vi "Check Notebook Status Before Quitting App.vi"(8 "Error In":errorcluster, 11 "App name":string) -> (0 "Error Out":errorcluster, 3 "Quit App?":bool)   [LabVIEW 2021, in "Notebook.lvlib"]
uses:
  Notebook.lvlib
  Notebook Parameters List.ctl
  Variant/Variant to Data/Variant to Data.lvlib
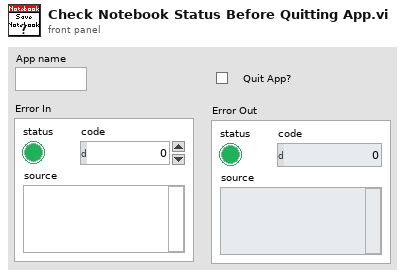
[diagram p1: front panel]
types:
  T1 = typedef "Notebook.lvlib/Notebook Parameters List.ctl" = enum16{"First Opening?", "Saved Notebook?", "Saved Notebook Path", "Beep on Error?"}
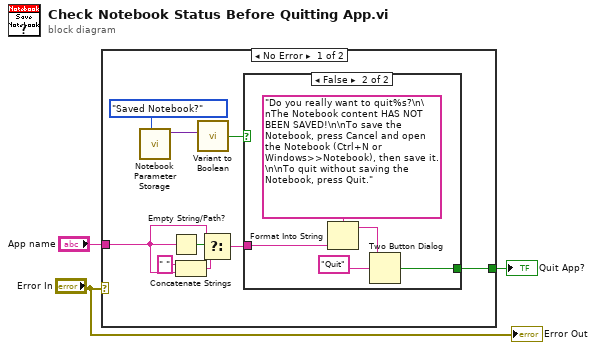
[diagram p0: block diagram]
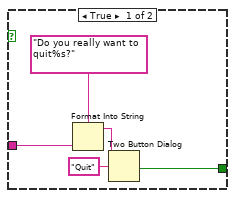
[diagram p2: hidden frame]
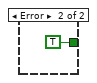
[diagram p3: hidden frame]
diagram:
  n1 = case shown="No Error" "Error In" {
    tunnel: "App name" -> [w8 _]
    tunnel: [w7 TRUE ("T button?")] -> w2
    frame No Error {
      n2 = call "Notebook Parameter Storage.vi"("Notebook Parameter List"=Notebook_Parameters_List."Saved Notebook?") -> ("Data out"=w6:variant)  [unwired: 9 in, 1 out]
      n3 = Empty String/Path?(string/path=w8) -> (empty?=w10:bool)
      n4 = Concatenate Strings(" " ("string"), w8) -> (w9:string)
      n5 = call "Variant to Boolean.vi"("Variant"=w6) -> ("Value"=w4:bool)  [unwired: 8 in]
      n6 = Select(t=w8, s=w10, f=w9) -> (s? t:f=w12:string)
      n7 = case shown="False" w4 {
        tunnel: [w15 w22] -> w7
        tunnel: w12 -> [w13 w18]
        frame True {
          n8 = Format Into String(format string="Do you really want to quit%s?" ("message"), w13) -> (resulting string=w14:string)  [unwired: 2 in, 1 out]
          n9 = Two Button Dialog(message=w14, 2:"Quit" ("T button name (\"OK\")")) -> (T button?=w15:bool)  [unwired: 1 in]
        }
        frame False {
          n10 = Format Into String(format string="Do you really want to quit%s?\n\nThe Notebook content HAS NOT BEEN SAVED!\n\nTo save the Notebook, press Cancel and open the Notebook (Ctrl+N or Windows>>Notebook), then save it.\n\nTo quit without saving the Notebook, press Quit." ("message"), w18) -> (resulting string=w19:string)  [unwired: 2 in, 1 out]
          n11 = Two Button Dialog(message=w19, 2:"Quit" ("T button name (\"OK\")")) -> (T button?=w22:bool)  [unwired: 1 in]
        }
      }
    }
    frame Error {
    }
  }
  "Quit App?" <- w2
  "Error Out" <- "Error In"
